vi "Correct Format String Position.vi"(8 "error in (no error)":errorcluster, 10 "format into string in":refnum<vi>, 11 "format string in":refnum<vi>) -> (0 "error out":errorcluster, 2 "format into string out":refnum<vi>, 3 "format string out":refnum<vi>)   [LabVIEW 2016]
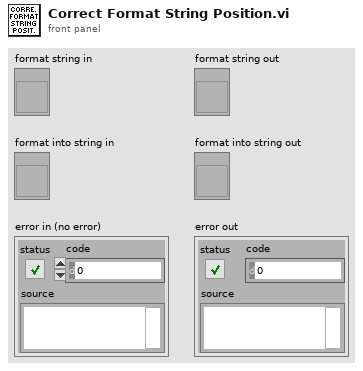
[diagram p1: front panel]
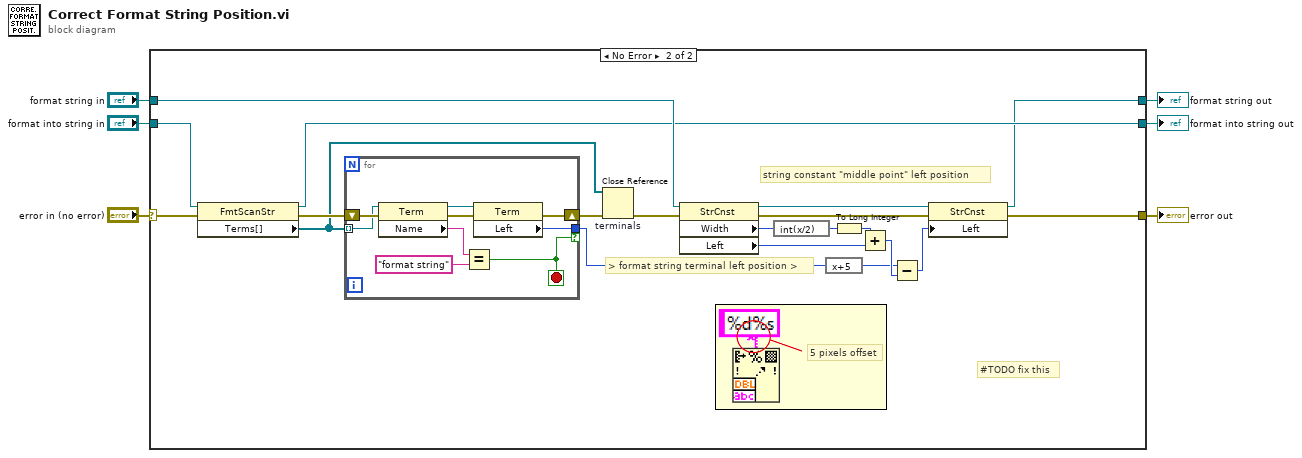
[diagram p0: block diagram]
diagram:
  n1 = case shown="No Error" "error in (no error)" {
    selector: "error in (no error)" -> [w9 w12]
    tunnel: "format string in" -> [w8 w21]
    tunnel: "format into string in" -> [w7 w18]
    tunnel: [w7 w17] -> w4
    tunnel: [w8 w16] -> w3
    tunnel: [w9 w13] -> w1
    frame Error {
    }
    frame No Error {
      # "#TODO fix this"
      # "string constant \"middle point\" left position"
      # "> format string terminal left position >"
      # "5 pixels offset"
      n2 = property class="FmtScanStr"(reference=w18, error in=w12) -> (reference out=w17:refnum<vi>, error out=w19:errorcluster, "Terms[]"=w14:refnum<vi>[])
      n3 = for {
        tunnel: w14 -> [w37] mode=indexing
        shift-right: [w30] -> w20
        shift-left: w19 -> [w38]
        tunnel: [w32] -> w11 if=w31
        stop <- w31 stop-if-true
        n4 = property class="Term"(reference=w37, error in=w38) -> (reference out=w34:refnum<vi>, error out=w33:errorcluster, "Name"=w36:string)
        n5 = Equal?(x=w36, y="format string") -> (x = y?=w31:bool)
        n6 = property class="Term"(reference=w34, error in=w33) -> (error out=w30:errorcluster, "Left"=w32:i32)  [unwired: 1 out]
      }
      n7 = Close Reference "terminals"(reference=w14, error in (no error)=w20) -> (error out=w15:errorcluster)
      n8 = property class="StrCnst"(reference=w21, error in=w15) -> (reference out=w22:refnum<vi>, error out=w23:errorcluster, "Width"=w24:u32, "Left"=w27:i32)
      n9 = expression code="int(x/2)"(w24) -> (w25:u32)
      n10 = expression code="x+5"(w11) -> (w10:i32)
      n11 = To Long Integer(number=w25) -> (32bit integer=w26:i32)
      n12 = Add(x=w26, y=w27) -> (x+y=w28:i32)
      n13 = Subtract(x=w10, y=w28) -> (x-y=w29:i32)
      n14 = property class="StrCnst"(reference=w22, error in=w23, "Left"=w29) -> (reference out=w16:refnum<vi>, error out=w13:errorcluster)
    }
  }
  "format into string out" <- w4
  "format string out" <- w3
  "error out" <- w1
